vi "GOMDBTS2048 substitution Geo Measurement With Test Device.vi"(8 "error in (no error)":errorcluster, 10 "isExternalSphere":bool, 11 "handle":i32) -> (0 "error out":errorcluster, 1 "current":dbl, 2 "counts":dbl[](array[numeric]), 3 "saturation":dbl, 5 "function return":i32)   [LabVIEW 2015, in "GOMDBTS2048.lvlib"]
doc: "GOBTS2048DLL int __stdcall GOMDBTS2048_substitutionMeasurementWithTestDevice(int handle, bool isExternalSphere, double* saturation, double* counts, double* current);"
uses:
  GOMDBTS2048.lvlib
  runtime/GOMDBTS2048.dll
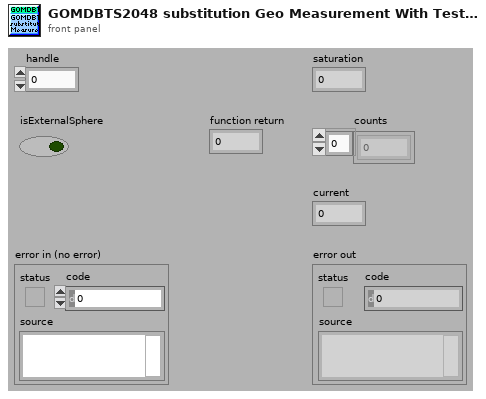
[diagram p1: front panel]
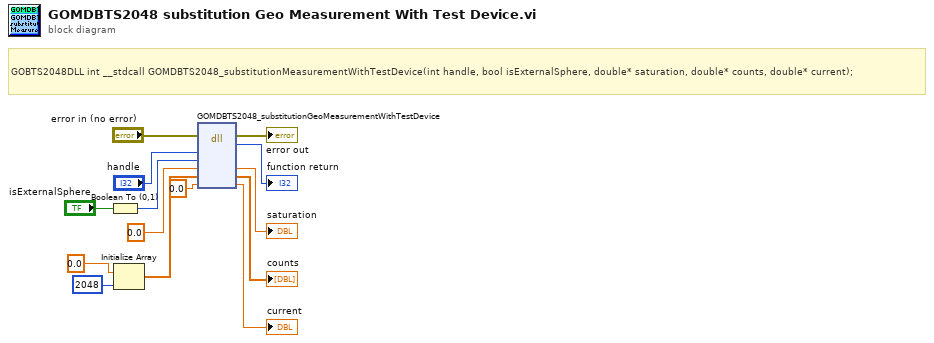
[diagram p0: block diagram]
diagram:
  # "GOBTS2048DLL int __stdcall GOMDBTS2048_substitutionMeasurementWithTestDevice(int handle, bool isExternalSphere, double* saturation, double* counts, double* current);"
  n1 = Boolean To (0,1)(Boolean="isExternalSphere") -> (0, 1=w11:i16)
  n2 = Initialize Array(0.0 ("element"), 2048 ("dimension size")) -> (w8:dbl[])
  n3 = dll-call lib="C:/Users/rkoch/Documents/GO_Library/runtime/GOMDBTS2048.*" fn="GOMDBTS2048_substitutionGeoMeasurementWithTestDevice"(error in="error in (no error)", "handle"="handle", "isExternalSphere"=w11, "saturation"=0.0, "counts"=w8, "current"=0.0) -> (error out=→"error out":errorcluster, "return type"=→"function return":i32, "saturation"=→"saturation":dbl, "counts"=→"counts":dbl[], "current"=→"current":dbl)  [unwired: 4 in, 1 out]
